vi "HFRR ADV v013 new software.vi"() -> ()   [LabVIEW 2025] (continued)
                              }
                              frame #3 {
                                n2582 = Wait (ms)(milliseconds to wait=u32 1500) -> ()  [unwired: 1 out]
                              }
                              frame #4 {
                                n2583 = local write "Command"("HE;0" ("Command")) -> ()
                              }
                            }
                          }
                        }
                      }
                      frame True {
                      }
                    }
                    n2584 = local write "String 14"("Test will autostart once parameters reach the set value." ("String 14")) -> ()
                  }
                  frame True {
                    (unwired) FALSE ("Visible")
                    n2585 = property on="Stroke 2" class="DigNum (strict)"("Visible"=TRUE) -> ()  [unwired: 2 in, 2 out]
                    n2586 = property on="STOP 2" class="Bool (strict)"("Disabled"=u8 2) -> ()  [unwired: 2 in, 2 out]
                    n2587 = local write "String 14"(" Running....." ("String 14")) -> ()
                    n2588 = property on="Heater Button" class="Bool (strict)"("DisabledEnum"=T17."Disabled and Grayed Out" ("Disabled")) -> ()  [unwired: 2 in, 2 out]
                    n2589 = property on="Humidity" class="Bool (strict)"("DisabledEnum"=T17."Disabled and Grayed Out" ("Disabled")) -> ()  [unwired: 2 in, 2 out]
                    n2590 = case shown="True" "Start Time" {
                      selector: "Start Time" -> [_ w3109]
                      frame False {
                      }
                      frame True {
                        n2591 = Not(x=w3109) -> (.not. x?=w3108:bool)
                        n2592 = local write "Start Time"(w3108) -> ()
                        n2593 = local read "EVENT LOG"() -> (w3110:string)
                        n2594 = call "Event Log.vi"("Content"="Test in progress", "EVENT LOG"=w3110) -> ("EVENT LOG"=w3112:string)  [unwired: 8 in, 1 out]
                        n2595 = local write "EVENT LOG"(w3112) -> ()
                      }
                    }
                    n2596 = disable-structure shown="Enabled" {
                      disable-tunnel: [w3101 w3107] -> w3090
                      frame Disabled {
                        n2597 = local read "Set Hz"() -> (w3104:dbl)
                        n2598 = call <vilib>:"Uniform White Noise Waveform.vi"() -> ("signal out"=w3103:waveform(dbl))  [unwired: 10 in, 1 out]
                        n2599 = Random Number (0-1)() -> (number: 0 to 1=w3100:dbl)
                        n2600 = Add(x=w3104, y=w3103) -> (x+y=w3102:waveform(dbl))
                        n2601 = Multiply(x=ext 0.01 ("y"), y=w3100) -> (x*y=w3098:ext)
                        n2602 = Multiply(x=w3102, y=w3098) -> (x*y=w3101:waveform(ext))
                      }
                      frame Enabled {
                        n2603 = call-poly <vilib>:"Random Number (Range).vi"("lower bound (0)"=49.89, "upper bound (100)"=50.8) -> ("number"=w3107:dbl)  [unwired: 9 in]
                      }
                    }
                    "StartFlg" <- TRUE ("StartFlg")
                  }
                }
                n2604 = case shown="True" w3061 {
                  frame False {
                  }
                  frame True {
                    n2605 = local write "clk"(10.0 ("clk")) -> ()
                    n2606 = Get Date/Time In Seconds() -> (seconds since 1Jan1904=w3115:timestamp)
                    n2607 = To Double Precision Float(number=w3115) -> (double precision float=w3113:dbl)
                    n2608 = local write "acq timer"(w3113) -> ()
                    n2609 = local write "act save time"(w3113) -> ()
                  }
                }
                n2610 = call "Elapsed Time"("Time Target (s)"="Countdown", "Reset"=w3050) -> ("Elapsed Time (s)"=w3055:dbl, "Time has Elapsed"=w3053:bool)  [unwired: 10 in, 6 out]
                "Countdown 2" <- w3055
                n2611 = Subtract(x=w3055, y=2.0) -> (x-y=w3058:dbl)
                n2612 = Less?(x=w3058, y="Countdown") -> (x < y?=w3056:bool)
                n2613 = And(x=w3056, y=w3053) -> (x .and. y?=w3052:bool)
                n2614 = case shown="True" w3052 {
                  frame False {
                  }
                  frame True {
                    (unwired) dbl[] [] ("History Data")
                    n2615 = local write "Engage"(FALSE ("Engage")) -> ()
                    n2616 = local write "RUN"(TRUE ("RUN")) -> ()
                    n2617 = local read "Humidity ( %RH )"() -> (→"Rh Before":dbl)
                  }
                }
                n2618 = local read "Test \nStatus"() -> (w3048:bool)
                n2619 = Select(t=w3046, s=w3048, f=0.0) -> (s? t:f=w3047:dbl)
                n2620 = local write "Frequency ( Hz )"(w3047) -> ()
              }
              frame #1 {
                w3138 = 1000000.0 ("x")
                # "HC;1/0\nST;VALUE"
                # "Elapsed time\ncof\nstroke\nAir temp\nTemp\nHumidity"
                # "acq timer\n\nact save time"
                # "convert to microseconds"
                n2621 = local read "COUNT"() -> (w3121:i32)
                n2622 = local read "Rate"() -> (w3134:dbl)
                n2623 = Divide(x=w3138, y=w3134) -> (x/y=w3139:dbl)
                n2624 = Greater Or Equal?(x=w3121, y=250) -> (x >= y?=w3120:bool)
                n2625 = Get Date/Time In Seconds() -> (seconds since 1Jan1904=w3141:timestamp)
                n2626 = case shown="True" w3120 {
                  frame False {
                    n2627 = local read "COUNT"() -> (w3142:i32)
                    n2628 = Increment(x=w3142) -> (x+1=w3143:i32)
                    n2629 = local write "COUNT"(w3143) -> ()
                  }
                  frame True {
                    n2630 = local write "COUNT"(0 ("COUNT")) -> ()
                  }
                }
                n2631 = local read "Samplingtime 2"() -> (w3119:dbl)
                n2632 = local read "act save time"() -> (w3136:dbl)
                n2633 = Divide(x=w3139, y=w3138) -> (x/y=w3137:dbl)
                n2634 = To Double Precision Float(number=w3141) -> (double precision float=w3130:dbl)
                n2635 = Add(x=w3136, y=w3119) -> (x+y=w3135:dbl)
                n2636 = local read "acq timer"() -> (w3140:dbl)
                n2637 = local read "COUNT"() -> (w3123:i32)
                n2638 = Greater Or Equal?(x=w3130, y=w3135) -> (x >= y?=w3118:bool)
                n2639 = Multiply(x=w3137, y=w3123) -> (x*y=w3129:dbl)
                n2640 = Subtract(x=w3130, y=w3140) -> (x-y=w3132:dbl)
                n2641 = local read "Save"() -> (w3133:bool)
                n2642 = Add(x=w3132, y=w3129) -> (x+y=w3116:dbl)
                "Elapsed time 3" <- w3116
                n2643 = And(x=w3118, y=w3133) -> (x .and. y?=w3131:bool)
                n2644 = Divide(x=w3116, y=60.0) -> (x/y=w3127:dbl)
                n2645 = local read "Test \nStatus"() -> (w3117:bool)
                n2646 = local read "clk"() -> (w3124:dbl)
                n2647 = Equal?(x=w3124, y=10.0) -> (x = y?=w3126:bool)
                n2648 = case shown="True" w3131 {
                  tunnel: w3130 -> [_ w3254]
                  tunnel: [FALSE ("Boolean 2") TRUE ("Boolean 2")] -> _
                  frame False {
                  }
                  frame True {
                    w3208 = ";" ("Substring")
                    # "Pid out/\nFreq response value"
                    n2649 = local write "act save time"(w3254) -> ()
                    n2650 = local read "FILE"() -> (w3202:string)
                    n2651 = call "file check.vi"("file name in"=w3202) -> ("error out"=w3205:errorcluster, "file name out"=w3200:string)  [unwired: 9 in]
                    n2652 = local read "LVDT STROKE"() -> (w3197:dbl)
                    n2653 = local read "Add up Stroke"() -> (w3195:dbl)
                    n2654 = call "FILE PATH CREATION.vi"("error in"=w3205, "FILE NAME :"=w3200) -> ("FILE OUT"=w3203:path)  [unwired: 8 in, 1 out]
                    n2655 = Concatenate Strings(w3200, ".dgf" ("Substring")) -> (w3204:string)
                    n2656 = Subtract(x=w3197, y=w3195) -> (x-y=w3196:dbl)
                    n2657 = Absolute Value(x=w3196) -> (abs(x)=w3194:dbl)
                    n2658 = local read "FF 2"() -> (→"Frictional Force ( N )" →"Frictional Force ( N )":dbl)
                    n2659 = Build Path(base path=w3203, name or relative path=w3204) -> (appended path=w3199:path)
                    n2660 = local read "COF 2"() -> (w3213:dbl)
                    "cof" <- w3213
                    "Coefficient of Friction" <- w3213
                    "COF 4" <- w3213
                    "Coefficient of Friction" <- w3213
                    n2661 = local read "TEMP"() -> (w3216:dbl)
                    "Temp" <- w3216
                    "Temperature ( Deg C )" <- w3216
                    n2662 = local read "Humidity ( %RH )"() -> (w3215:dbl)
                    "Humidity ( %RH )" <- w3215
                    "Humidity ( %RH )" <- w3215
                    n2663 = local read "Frequency ( Hz )"() -> (w3222:dbl)
                    n2664 = call <vilib>:"Mean PtByPt.vi"("x"=w3194, "sample length"=10) -> ("mean"=w3193:dbl)  [unwired: 2 in, 1 out]
                    n2665 = local read "Elapsed time"() -> (w3247:dbl)
                    n2666 = local read "AIR TEMP"() -> (w3220:dbl)
                    n2667 = local read "PID-out"() -> (w3225:dbl)
                    n2668 = local write "Temperature ( Deg C )"(w3216) -> ()
                    n2669 = Number To Fractional String(number=w3193, width (-)=i16 9 ("precision (6)"), precision (6)=i16 6) -> (F-format string=w3240:string)  [unwired: 1 in]
                    n2670 = Number To Fractional String(number=w3220, width (-)=i16 9 ("precision (6)"), precision (6)=i16 3) -> (F-format string=w3239:string)  [unwired: 1 in]
                    n2671 = Number To Fractional String(number=w3216, width (-)=i16 9 ("precision (6)"), precision (6)=i16 3) -> (F-format string=w3236:string)  [unwired: 1 in]
                    n2672 = Number To Fractional String(number=w3215, width (-)=i16 9 ("precision (6)"), precision (6)=i16 3) -> (F-format string=w3233:string)  [unwired: 1 in]
                    n2673 = Number To Fractional String(number=0.0, width (-)=i16 9 ("precision (6)"), precision (6)=i16 3) -> (F-format string=w3230:string)  [unwired: 1 in]
                    n2674 = Number To Fractional String(number=w3225, width (-)=i16 9 ("precision (6)"), precision (6)=i16 3) -> (F-format string=w3226:string)  [unwired: 1 in]
                    n2675 = Number To Fractional String(number=w3222, width (-)=i16 9 ("precision (6)"), precision (6)=i16 3) -> (F-format string=w3221:string)  [unwired: 1 in]
                    n2676 = Number To Fractional String(number=w3213, width (-)=i16 9 ("precision (6)"), precision (6)=i16 6) -> (F-format string=w3248:string)  [unwired: 1 in]
                    n2677 = Number To Fractional String(number=w3247, width (-)=i16 14 ("precision (6)"), precision (6)=i16 3) -> (F-format string=w3249:string)  [unwired: 1 in]
                    n2678 = Bundle("y"=1.02, "mean"=w3193, "y"=0.98) -> (w3214:cluster{"y":dbl, "mean":dbl, "y":dbl})  [unwired: 1 in]
                    n2679 = Number To Fractional String(number="Ambient Humidity :", width (-)=i16 9 ("precision (6)"), precision (6)=i16 6) -> (F-format string=w3206:string)  [unwired: 1 in]
                    n2680 = local read "RUN"() -> (w3212:bool)
                    n2681 = case shown="True" w3212 {
                      tunnel: w3214 -> [_ w3259]
                      tunnel: w3193 -> [_ w3258]
                      tunnel: w3193 -> [_ w3256]
                      tunnel: w3193 -> [_ w3257]
                      frame False {
                      }
                      frame True {
                        "Stroke ( mm )" <- w3259
                        "Stroke ( mm )" <- w3259
                        "Stroke 4" <- w3258
                        "Stroke 3" <- w3256
                        "Stroke 2" <- w3257
                        "measured_stroke" <- w3256
                      }
                    }
                    n2682 = Concatenate Strings(w3249, w3208, w3248, w3208, w3240, w3208, w3239, w3208, w3236, w3208, w3233, w3208, w3230, w3208, w3226, w3208, w3221, w3208, w3206, "\r") -> (w3246:string)
                    n2683 = call <vilib>:"Write Characters To File.vi"("append to file? (new file:F)"=TRUE, "character string"=w3246, "file path (dialog if empty)"=w3199) -> ()  [unwired: 2 in, 1 out]
                    "refresh flag" <- TRUE ("refresh flag")
                  }
                }
                n2684 = case shown="True" w3117 {
                  tunnel: w3127 -> [_ w3153]
                  tunnel: w3132 -> [_ w3163]
                  tunnel: [0.0 w3159] -> _
                  tunnel: w3126 -> [_ w3158]
                  tunnel: [0.0 w3157] -> _
                  tunnel: w3116 -> [_ w3157]
                  tunnel: w3130 -> [w3146 _]
                  frame False {
                    n2685 = local write "acq timer"(w3146) -> ()
                    n2686 = local write "Test Duration Status"(0.0 ("Test Duration Status")) -> ()
                  }
                  frame True {
                    n2687 = local read "Set Hz"() -> (w3160:dbl)
                    n2688 = local write "Elapsed time"(w3153) -> ()
                    n2689 = local read "test time"() -> (w3152:dbl)
                    n2690 = Multiply(x=w3163, y=w3160) -> (x*y=w3162:dbl)
                    n2691 = case shown="False" w3158 {
                      tunnel: w3162 -> [w3164 _]
                      tunnel: [w3164 1.0] -> w3159
                      frame False {
                        n2692 = local write "Cycles elapsed"(w3164) -> ()
                      }
                      frame True {
                      }
                    }
                    n2693 = Greater?(x=w3153, y=w3152) -> (0:w3161:bool)
                    n2694 = Subtract(x=w3152, y=w3153) -> (x-y=w3151:dbl)
                    "time" <- w3151
                    n2695 = Multiply(x=w3151, y=60.0) -> (x*y=w3150:dbl)
                    n2696 = local write "Time Remaining"(w3150) -> ()
                    n2697 = local write "Remaining Time"(w3150) -> ()
                    n2698 = case shown="True" w3161 {
                      frame False {
                      }
                      frame True {
                        n2699 = stacked-sequence {
                          frame #0 {
                            w3169 = T17."Enabled" ("Disabled")
                            w3168 = FALSE ("TEST FILE NAM,E SAVED")
                            w3170 = "" ("FILE")
                            w3171 = TRUE ("Visible")
                            n2700 = local write "Humidity"(FALSE ("Humidity")) -> ()
                            n2701 = local write "RUN"(FALSE ("OK Button 2")) -> ()
                            n2702 = local write "Heater Button"(FALSE ("Heater Button")) -> ()
                            n2703 = local write "Auto Start Test"(FALSE ("Auto Start Test")) -> ()
                            n2704 = local write "TestCompFlg"(TRUE ("StpFlg")) -> ()
                            n2705 = local read "Humidity ( %RH )"() -> (→"Rh After":dbl)
                            n2706 = property on="STOP 2" class="Bool (strict)"("Disabled"=u8 0) -> ()  [unwired: 2 in, 2 out]
                            n2707 = local read "EVENT LOG"() -> (w3176:string)
                            n2708 = call "Event Log.vi"("Content"="Test Completed", "EVENT LOG"=w3176) -> ("EVENT LOG"=w3175:string)  [unwired: 8 in, 1 out]
                            n2709 = property on="RUN" class="Bool (strict)"("Visible"=w3171) -> ()  [unwired: 2 in, 2 out]
                            n2710 = property on="Auto Start Test" class="Bool (strict)"("Visible"=w3171) -> ()  [unwired: 2 in, 2 out]
                            n2711 = local write "Batch Ref Num :"(w3170) -> ()
                            n2712 = local write "FILE"(w3170) -> ()
                            n2713 = local write "EVENT LOG"(w3175) -> ()
                            n2714 = local write "TEST FILE NAM,E SAVED"(w3168) -> ()
                            n2715 = local write "Fuel Discription :"(w3170) -> ()
                            n2716 = local write "START TEMP"(w3168) -> ()
                            n2717 = local write "Remarks :"(w3170) -> ()
                            n2718 = local write "Main Dashboard Buttons"(T1."Imaging" ("Main Dashboard Buttons")) -> ()
                            n2719 = local write "Main Tab"(T2."Adv Scar" ("Main Tab")) -> ()
                            n2720 = property on="FRICVALZ 2" class="Bool (strict)"("DisabledEnum"=w3169) -> ()  [unwired: 2 in, 2 out]
                            n2721 = property on="FRICVALZ 3" class="Bool (strict)"("DisabledEnum"=w3169) -> ()  [unwired: 2 in, 2 out]
                            n2722 = property on="FRICVALZ 4" class="Bool (strict)"("DisabledEnum"=w3169) -> ()  [unwired: 2 in, 2 out]
                          }
                          frame #1 {
                            n2723 = Wait (ms)(milliseconds to wait=u32 1500) -> ()  [unwired: 1 out]
                          }
                          frame #2 {
                            n2724 = local write "Command"("VC;0") -> ()
                          }
                          frame #3 {
                            n2725 = Wait (ms)(milliseconds to wait=u32 1500) -> ()  [unwired: 1 out]
                          }
                          frame #4 {
                            n2726 = local write "Command"("VC;0") -> ()
                          }
                          frame #5 {
                            n2727 = Wait (ms)(milliseconds to wait=u32 1500) -> ()  [unwired: 1 out]
                          }
                          frame #6 {
                            n2728 = local write "Command"("ST;0") -> ()
                          }
                          frame #7 {
                            n2729 = local write "measured_stroke"(0.0 ("measured_stroke")) -> ()
                            n2730 = Wait (ms)(milliseconds to wait=u32 1500) -> ()  [unwired: 1 out]
                          }
                          frame #8 {
                            n2731 = local write "Command"("HE;0") -> ()
                          }
                        }
                      }
                    }
                    n2732 = Divide(x=w3153, y=w3152) -> (x/y=w3156:dbl)
                    n2733 = Multiply(x=w3156, y=100.0) -> (x*y=w3154:dbl)
                    n2734 = local write "Test Duration Status"(w3154) -> ()
                  }
                }
              }
              frame #2 {
                n2735 = case shown="True" "Heater Button" {
                  tunnel: [0.0 ("output") w3282] -> w3260
                  frame False {
                    w3263 = TRUE ("tmpchk")
                    n2736 = local read "TEMP"() -> (w3264:dbl)
                    n2737 = local write "Temp ini"(w3264) -> ()
                    n2738 = local write "Reset 4"(w3263) -> ()
                    n2739 = local write "tmpchk"(w3263) -> ()
                    n2740 = local write "reinit"(TRUE ("reinit")) -> ()
                    n2741 = local write "manual temp log"(TRUE ("manual temp log")) -> ()
                  }
                  frame True {
                    # "Logic to turn off\nthe heater when \ntemp is not rising.\nTime - 60 sec\nDelta t- 5°c"
                    n2742 = local read "Temp ini"() -> (w3271:dbl)
                    n2743 = local read "Auto Start Test"() -> (w3267:bool)
                    n2744 = Less?(x=w3271, y=53.0) -> (x < y?=w3269:bool)
                    n2745 = case shown="False" w3267 {
                      frame False {
                        n2746 = local read "Set Temp"() -> (w3291:dbl)
                        n2747 = local read "TEMP"() -> (w3290:dbl)
                        n2748 = Subtract(x=w3291, y=w3290) -> (x-y=w3289:dbl)
                        n2749 = Absolute Value(x=w3289) -> (abs(x)=w3288:dbl)
                        n2750 = Less?(x=w3288, y=0.5) -> (x < y?=w3286:bool)
                        n2751 = case shown="True" w3286 {
                          tunnel: "manual temp log" -> [_ w3292]
                          frame False {
                          }
                          frame True {
                            n2752 = case shown="True" w3292 {
                              selector: w3292 -> [_ w3293]
                              frame False {
                              }
                              frame True {
                                # "#Event log"
                                n2753 = Not(x=w3293) -> (.not. x?=w3294:bool)
                                n2754 = local write "manual temp log"(w3294) -> ()
                                n2755 = local read "EVENT LOG"() -> (w3297:string)
                                n2756 = call "Event Log.vi"("Content"="Target Temperature reached", "EVENT LOG"=w3297) -> ("EVENT LOG"=w3296:string)  [unwired: 8 in, 1 out]
                                n2757 = local write "EVENT LOG"(w3296) -> ()
                              }
                            }
                          }
                        }
                      }
                      frame True {
                        n2758 = local write "manual temp log"(TRUE ("manual temp log")) -> ()
                      }
                    }
                    n2759 = And(x="tmpchk", y=w3269) -> (x .and. y?=w3272:bool)
                    n2760 = case shown="True" w3272 {
                      frame False {
                      }
                      frame True {
                        n2761 = call "Elapsed Time8"("Time Target (s)"=300.0, "Reset"="Reset 4") -> ("Time has Elapsed"=w3299:bool)  [unwired: 10 in, 7 out]
                        n2762 = flat-sequence {
                          tunnel: w3299 -> [_]
                          frame #0 {
                            n2763 = local write "Reset 4"(FALSE ("Reset 4")) -> ()
                          }
                        }
                        n2764 = case shown="True" w3299 {
                          frame False {
                          }
                          frame True {
                            n2765 = local read "Temp ini"() -> (w3306:dbl)
                            n2766 = Add(x=w3306, y=5.0) -> (x+y=w3304:dbl)
                            n2767 = local read "TEMP"() -> (w3307:dbl)
                            n2768 = Greater?(x=w3307, y=w3304) -> (0:w3305:bool)
                            n2769 = case shown="False" w3305 {
                              frame False {
                                n2770 = local write "Heater Button"(FALSE ("Heater Button")) -> ()
                              }
                              frame True {
                                n2771 = local write "tmpchk"(FALSE ("tmpchk")) -> ()
                              }
                            }
                          }
                        }
                      }
                    }
                    n2772 = local read "Set Temp"() -> (w3280:dbl)
                    n2773 = local read "TEMP"() -> (w3274:dbl)
                    n2774 = call-poly <vilib>:"PID.vi"("reinitialize? (F)"="reinit", "dt (s)"=-1.0, "process variable"=w3274, "setpoint"=w3280) -> ("output"=w3277:dbl)  [unwired: 6 in, 1 out]
                    n2775 = Subtract(x=w3280, y=w3274) -> (x-y=w3281:dbl)
                    n2776 = Add(x=w3280, y=0.5) -> (x+y=w3278:dbl)
                    n2777 = Greater Or Equal?(x=w3274, y=w3278) -> ()  [unwired: 1 out]
                    n2778 = Select(t=0.0, s=FALSE, f=w3277) -> (s? t:f=w3276:dbl)
                    "PID output" <- w3276
                    n2779 = flat-sequence {
                      tunnel: w3276 -> [w3310]
                      tunnel: [w3310] -> w3282
                      frame #0 {
                        n2780 = local write "reinit"(FALSE ("reinit")) -> ()
                      }
                    }
                    n2781 = Bundle(w3281, "output"=w3276, "TEMP"=w3274) -> ()  [unwired: 1 in, 1 out]
                  }
                }
                "PID-out" <- w3260
              }
              frame #3 {
                n2782 = local read "TEMP"() -> (w3312:dbl)
                n2783 = Greater Or Equal?(x=w3312, y="Set Temp 2") -> (x >= y?=w3317:bool)
                n2784 = case shown="True" w3317 {
                  tunnel: [FALSE TRUE] -> w3315
                  frame False {
                  }
                  frame True {
                  }
                }
                "Status 13" <- w3315
                n2785 = And(x=w3315, y="trip1 8") -> (x .and. y?=w3314:bool)
                n2786 = case shown="True" w3314 {
                  frame False {
                    n2787 = local write "Heater Trip Temp"(TRUE ("Heater Trip Temp")) -> ()
                  }
                  frame True {
                    w3320 = FALSE ("OK Button 2")
                    n2788 = case shown="True" "Heater Trip Temp" {
                      selector: "Heater Trip Temp" -> [_ w3322]
                      frame False {
                      }
                      frame True {
                        n2789 = Not(x=w3322) -> (.not. x?=w3321:bool)
                        n2790 = local read "EVENT LOG"() -> (w3325:string)
                        n2791 = local write "Heater Trip Temp"(w3321) -> ()
                        n2792 = call "Event Log.vi"("Content"="Heater Trip", "EVENT LOG"=w3325) -> ("EVENT LOG"=w3324:string)  [unwired: 8 in, 1 out]
                        n2793 = local write "EVENT LOG"(w3324) -> ()
                      }
                    }
                    n2794 = local write "RUN"(w3320) -> ()
                    n2795 = property on="Auto Start Test" class="Bool (strict)"("Value"=w3320) -> ()  [unwired: 2 in, 2 out]
                    n2796 = local write "Heater Button"(w3320) -> ()
                  }
                }
              }
            }
            n2797 = case shown="False" w3041 {
              frame False {
                n2798 = disable-structure shown="Disabled" {
                  frame Disabled {
                    n2799 = stacked-sequence {
                      frame #0 {
                        n2800 = local write "RUN"(FALSE ("OK Button 2")) -> ()
                      }
                      frame #1 {
                      }
                    }
                  }
                  frame Enabled {
                  }
                }
              }
              frame True {
              }
            }
          }
        }
        n2801 = local read "airtempflg"() -> (w2833:bool)
        n2802 = Or(x=w2833, y=w2831) -> (x .or. y?=w2834:bool)
        n2803 = Insert Into Array(array=string[] ["Air Temperature has reached set value,", "Humidity has reached set value,", "Sample Temperaturehas reached set value,", ""], index=0, new element="") -> (w2819:string[])
        n2804 = Build Array(w2824, w2823, w2822) -> (w2820:i32[])
        n2805 = disable-structure shown="Disabled" {
          disable-tunnel: w2834 -> [w2911 _]
          disable-tunnel: w2829 -> [w2910 _]
          disable-tunnel: w2827 -> [w2909 _]
          frame Disabled {
            n2806 = Compound Arithmetic op=AND(w2911, w2910, w2909) -> ()  [unwired: 1 out]
            n2807 = case shown="True" {
              selector: _ -> [_ _]
              frame False {
              }
              frame True {
                w2912 = FALSE ("autostrtflg")
                n2808 = local write "RUN"(TRUE ("RUN")) -> ()
                n2809 = local write "autostrtflg"(w2912) -> ()
                n2810 = local write "autostart"(w2912) -> ()
                n2811 = local write "String 14"(" Running....." ("String 14")) -> ()
              }
            }
          }
          frame Enabled {
          }
        }
        n2812 = for {
          tunnel: w2820 -> [w2962] mode=indexing
          tunnel: w2819 -> [w2961]
          shift-right: [w2958] -> w2818
          shift-left: "" -> [w2960]
          n2813 = Index Array(array=w2961, index=w2962) -> (element=w2959:string)
          n2814 = Concatenate Strings(w2959, w2960) -> (w2958:string)
        }
        n2815 = local write "autostart 2"(w2818) -> ()
        n2816 = local read "Reset Graph"() -> (w2807:bool)
        n2817 = case shown="True" w2807 {
          selector: w2807 -> [_ w2861]
          frame False {
          }
          frame True {
            w2875 = 0.0 ("X Scale.Range:Maximum")
            n2818 = Not(x=w2861) -> (.not. x?=w2860:bool)
            n2819 = local write "Reset Graph"(w2860) -> ()
            n2820 = property on="Electrical Contact Resistance ( % )" class="WFChart (strict)"("XScale.Maximum"=600.0 ("X Scale.Range:Maximum"), "XScale.Minimum"=0.0 ("X Scale.Range:Minimum"), "YScale.Maximum"=100.0 ("Y Scale.Range:Maximum"), "YScale.Minimum"=0.0 ("Y Scale.Range:Minimum")) -> ()  [unwired: 2 in, 2 out]
            n2821 = property on="Frictional Force ( N )" class="WFChart (strict)"("XScale.Maximum"=600.0 ("X Scale.Range:Maximum"), "XScale.Minimum"=0.0 ("X Scale.Range:Minimum"), "YScale.Maximum"=100.0 ("Y Scale.Range:Maximum"), "YScale.Minimum"=0.0 ("Y Scale.Range:Minimum")) -> ()  [unwired: 2 in, 2 out]
            n2822 = property on="Temperature ( Deg C )" class="WFChart (strict)"("XScale.Maximum"=600.0 ("X Scale.Range:Maximum"), "XScale.Minimum"=0.0 ("X Scale.Range:Minimum"), "YScale.Maximum"=100.0 ("Y Scale.Range:Maximum"), "YScale.Minimum"=0.0 ("Y Scale.Range:Minimum")) -> ()  [unwired: 2 in, 2 out]
            n2823 = property on="Humidity ( %RH )" class="WFChart (strict)"("XScale.Maximum"=600.0 ("X Scale.Range:Maximum"), "XScale.Minimum"=0.0 ("X Scale.Range:Minimum"), "YScale.Maximum"=100.0 ("Y Scale.Range:Maximum"), "YScale.Minimum"=0.0 ("Y Scale.Range:Minimum")) -> ()  [unwired: 2 in, 2 out]
            n2824 = property on="Stroke ( mm )" class="WFChart (strict)"("XScale.Maximum"=600.0 ("X Scale.Range:Maximum"), "XScale.Minimum"=0.0 ("X Scale.Range:Minimum"), "YScale.Maximum"=100.0 ("Y Scale.Range:Maximum"), "YScale.Minimum"=0.0 ("Y Scale.Range:Minimum")) -> ()  [unwired: 2 in, 2 out]
            n2825 = property on="Coefficient of Friction" class="WFChart (strict)"("XScale.Maximum"=600.0 ("X Scale.Range:Maximum"), "XScale.Minimum"=0.0 ("X Scale.Range:Minimum"), "YScale.Maximum"=100.0 ("Y Scale.Range:Maximum"), "YScale.Minimum"=0.0 ("Y Scale.Range:Minimum")) -> ()  [unwired: 2 in, 2 out]
            n2826 = property on="Electrical Contact Resistance ( % )" class="WFChart (strict)"("XScale.Minimum"=0.0 ("X Scale.Range:Minimum"), "XScale.Maximum"=600.0 ("X Scale.Range:Maximum"), "YScale.Minimum"=0.0 ("Y Scale.Range:Minimum"), "YScale.Maximum"=100.0 ("Y Scale.Range:Maximum")) -> ()  [unwired: 2 in, 2 out]
            n2827 = property on="Temperature ( Deg C )" class="WFChart (strict)"("XScale.Minimum"=0.0 ("X Scale.Range:Minimum"), "XScale.Maximum"=600.0 ("X Scale.Range:Maximum"), "YScale.Minimum"=0.0 ("Y Scale.Range:Minimum"), "YScale.Maximum"=100.0 ("Y Scale.Range:Maximum")) -> ()  [unwired: 2 in, 2 out]
            n2828 = property on="Coefficient of Friction" class="WFChart (strict)"("XScale.Minimum"=0.0 ("X Scale.Range:Minimum"), "XScale.Maximum"=600.0 ("X Scale.Range:Maximum"), "YScale.Maximum"=1.0 ("X Scale.Range:Minimum"), "YScale.Minimum"=0.0 ("X Scale.Range:Minimum")) -> ()  [unwired: 2 in, 2 out]
            n2829 = property on="Frictional Force ( N )" class="WFChart (strict)"("XScale.Maximum"=600.0 ("X Scale.Range:Maximum"), "XScale.Minimum"=w2875, "YScale.Maximum"=10.0 ("Y Scale.Range:Maximum"), "YScale.Minimum"=w2875) -> ()  [unwired: 2 in, 2 out]
            n2830 = property on="Stroke ( mm )" class="WFChart (strict)"("XScale.Maximum"=600.0 ("X Scale.Range:Maximum"), "XScale.Minimum"=0.0 ("X Scale.Range:Minimum"), "YScale.Maximum"=100.0 ("Y Scale.Range:Maximum"), "YScale.Minimum"=0.0 ("Y Scale.Range:Minimum")) -> ()  [unwired: 2 in, 2 out]
            n2831 = property on="Humidity ( %RH )" class="WFChart (strict)"("XScale.Maximum"=600.0 ("X Scale.Range:Maximum"), "XScale.Minimum"=0.0 ("X Scale.Range:Minimum"), "YScale.Maximum"=100.0 ("Y Scale.Range:Maximum"), "YScale.Minimum"=0.0 ("Y Scale.Range:Minimum")) -> ()  [unwired: 2 in, 2 out]
          }
        }
      }
      frame "Compare Files" {
        # "Elapsed time\ncof\nstroke\nAir temp\nTemp\nHumidity"
        n2832 = case shown="True" "RSTV1 2" {
          frame False {
          }
          frame True {
            n2833 = property on="Humidity ( %RH )" class="XYGraph (strict)"("Y Scale.Display Format:Precision"=u8 0 ("Y Scale.Format & Precision:Precision")) -> ()  [unwired: 2 in, 2 out]
            n2834 = property on="Humidity ( %RH )" class="XYGraph (strict)"("X Scale.Range:Minimum"=0.0, "X Scale.Range:Maximum"=75.0, "Y Scale.Range:Minimum"=48.0, "Y Scale.Range:Maximum"=58.0) -> ()  [unwired: 2 in, 2 out]
          }
        }
        n2835 = case shown="True" "RST CP 2" {
          frame False {
          }
          frame True {
            n2836 = property on="XY Graph 13" class="XYGraph (strict)"("Y Scale.Display Format:Precision"=u8 0 ("Y Scale.Format & Precision:Precision")) -> ()  [unwired: 2 in, 2 out]
            n2837 = property on="XY Graph 13" class="XYGraph (strict)"("X Scale.Range:Minimum"=0.0, "X Scale.Range:Maximum"=75.0, "Y Scale.Range:Minimum"=0.0, "Y Scale.Range:Maximum"=100.0) -> ()  [unwired: 2 in, 2 out]
          }
        }
        n2838 = case shown="True" "RST CP" {
          frame False {
          }
          frame True {
            n2839 = property on="Sample Temperature ( °C )" class="XYGraph (strict)"("Y Scale.Display Format:Precision"=u8 2 ("Y Scale.Format & Precision:Precision")) -> ()  [unwired: 2 in, 2 out]
            n2840 = property on="Sample Temperature ( °C )" class="XYGraph (strict)"("X Scale.Range:Minimum"=0.0, "X Scale.Range:Maximum"=75.0, "Y Scale.Range:Minimum"=58.0, "Y Scale.Range:Maximum"=62.0) -> ()  [unwired: 2 in, 2 out]
          }
        }
        n2841 = case shown="True" "RSTV1 3" {
          frame False {
          }
          frame True {
            n2842 = property on="Air Temperature  ( °C )" class="XYGraph (strict)"("Y Scale.Display Format:Precision"=u8 2 ("Y Scale.Format & Precision:Precision")) -> ()  [unwired: 2 in, 2 out]
            n2843 = property on="Air Temperature  ( °C )" class="XYGraph (strict)"("X Scale.Range:Minimum"=0.0 ("Y Scale.Range:Minimum"), "X Scale.Range:Maximum"=75.0 ("Y Scale.Range:Maximum"), "Y Scale.Range:Minimum"=20.0 ("X Scale.Range:Minimum"), "Y Scale.Range:Maximum"=26.0 ("X Scale.Range:Maximum")) -> ()  [unwired: 2 in, 2 out]
          }
        }
        n2844 = case shown="True" "RSTV1 4" {
          frame False {
          }
          frame True {
            n2845 = property on="Stroke ( mm )" class="XYGraph (strict)"("Y Scale.Display Format:Precision"=u8 2 ("Y Scale.Format & Precision:Precision")) -> ()  [unwired: 2 in, 2 out]
            n2846 = property on="Stroke ( mm )" class="XYGraph (strict)"("X Scale.Range:Minimum"=0.0 ("Y Scale.Range:Maximum"), "X Scale.Range:Maximum"=75.0 ("X Scale.Range:Minimum"), "Y Scale.Range:Minimum"=0.98, "Y Scale.Range:Maximum"=1.02) -> ()  [unwired: 2 in, 2 out]
          }
        }
        n2847 = case shown="True" "rstv2" {
          frame False {
          }
          frame True {
            n2848 = property on="Coefficient Of Friction" class="XYGraph (strict)"("Y Scale.Display Format:Precision"=u8 3 ("Y Scale.Format & Precision:Precision")) -> ()  [unwired: 2 in, 2 out]
            n2849 = property on="Coefficient Of Friction" class="XYGraph (strict)"("X Scale.Range:Minimum"=0.0 ("Y Scale.Range:Maximum"), "X Scale.Range:Maximum"=75.0, "Y Scale.Range:Minimum"=0.0, "Y Scale.Range:Maximum"=1.0 ("X Scale.Range:Minimum")) -> ()  [unwired: 2 in, 2 out]
          }
        }
        n2850 = case shown="True" "RST CP 3" {
          frame False {
          }
          frame True {
            n2851 = property on="Air Temp ( °C ) vs Humidity ( % RH )" class="XYGraph (strict)"("X Scale.Range:Minimum"=18.0, "X Scale.Range:Maximum"=28.0 ("X Scale.Range:Minimum"), "Y Scale.Range:Minimum"=30.0 ("X Scale.Range:Minimum"), "Y Scale.Range:Maximum"=70.0 ("X Scale.Range:Minimum")) -> ()  [unwired: 2 in, 2 out]
          }
        }
        n2852 = case shown="True" "OPEN 1" {
          frame False {
          }
          frame True {
            (unwired) 0  # existing file
            w3601 = "Choose a datalog file to open"  # prompt
            n2853 = local write "OPEN 1"(FALSE ("OPEN 1")) -> ()
            n2854 = String To Path(string="C:\\LAB-IQ\\Data\\") -> (path=w3586:path)
            n2855 = File Dialog(6:"*.dgf" ("pattern"), 7:w3601, 11:w3586) -> (0:w3584:errorcluster, 3:w3592:path)  [unwired: 4 in, 2 out]
            n2856 = Unbundle(w3584) -> ()  [unwired: 3 out]
            n2857 = Strip Path(path=w3592) -> (name=w3591:string)  [unwired: 1 out]
            n2858 = Path To String(path=w3592) -> (string=w3587:string)
            "string1" <- w3587
            n2859 = Match Pattern(string=w3591, regular expression=".dgf") -> (before substring=→"String Control":string)  [unwired: 1 in, 3 out]
            n2860 = Match Pattern(string=w3587, regular expression=".dgf" ("substring (\"\")")) -> (before substring=w3597:string)  [unwired: 1 in, 3 out]
            n2861 = Concatenate Strings(w3597, ".duf" ("Substring")) -> (w3593:string)
            n2862 = String To Path(string=w3593) -> (path=w3598:path)
            n2863 = call <vilib>:"Read Characters From File.vi"("file path (dialog if empty)"=w3598, "start of read offset (chars.:0)"=60 ("start of read offset (chars.: 0)")) -> ("character string"=→"String Control 2":string)  [unwired: 4 in, 3 out]
          }
        }
        n2864 = case shown="True" "OPEN 2" {
          frame False {
          }
          frame True {
            (unwired) 0  # existing file
            w3619 = "Choose a datalog file to open"  # prompt
            n2865 = local write "OPEN 2"(FALSE ("OPEN 1")) -> ()
            n2866 = String To Path(string="C:\\LAB-IQ\\Data\\") -> (path=w3604:path)
            n2867 = File Dialog(6:"*.dgf" ("pattern"), 7:w3619, 11:w3604) -> (0:w3602:errorcluster, 3:w3610:path)  [unwired: 4 in, 2 out]
            n2868 = Unbundle(w3602) -> ()  [unwired: 3 out]
            n2869 = Strip Path(path=w3610) -> (name=w3608:string)  [unwired: 1 out]
            n2870 = Path To String(path=w3610) -> (string=w3605:string)
            "string1 2" <- w3605
            n2871 = Match Pattern(string=w3608, regular expression=".dgf") -> (before substring=→"String Control 3":string)  [unwired: 1 in, 3 out]
            n2872 = Match Pattern(string=w3605, regular expression=".dgf" ("substring (\"\")")) -> (before substring=w3616:string)  [unwired: 1 in, 3 out]
            n2873 = Concatenate Strings(w3616, ".duf" ("Substring")) -> (w3613:string)
            n2874 = String To Path(string=w3613) -> (path=w3611:path)
            n2875 = call <vilib>:"Read Characters From File.vi"("file path (dialog if empty)"=w3611, "start of read offset (chars.:0)"=60 ("start of read offset (chars.: 0)")) -> ("character string"=→"String Control 4":string)  [unwired: 4 in, 3 out]
          }
        }
        n2876 = case shown="True" "OPEN 3" {
          frame False {
          }
          frame True {
            (unwired) 0  # existing file
            w3637 = "Choose a datalog file to open"  # prompt
            n2877 = local write "OPEN 3"(FALSE ("OPEN 1")) -> ()
            n2878 = String To Path(string="C:\\LAB-IQ\\Data\\") -> (path=w3622:path)
            n2879 = File Dialog(6:"*.dgf" ("pattern"), 7:w3637, 11:w3622) -> (0:w3620:errorcluster, 3:w3628:path)  [unwired: 4 in, 2 out]
            n2880 = Unbundle(w3620) -> ()  [unwired: 3 out]
            n2881 = Strip Path(path=w3628) -> (name=w3626:string)  [unwired: 1 out]
            n2882 = Path To String(path=w3628) -> (string=w3623:string)
            "string1 3" <- w3623
            n2883 = Match Pattern(string=w3626, regular expression=".dgf") -> (before substring=→"String Control 5":string)  [unwired: 1 in, 3 out]
            n2884 = Match Pattern(string=w3623, regular expression=".dgf" ("substring (\"\")")) -> (before substring=w3633:string)  [unwired: 1 in, 3 out]
            n2885 = Concatenate Strings(w3633, ".duf" ("Substring")) -> (w3630:string)
            n2886 = String To Path(string=w3630) -> (path=w3634:path)
            n2887 = call <vilib>:"Read Characters From File.vi"("file path (dialog if empty)"=w3634, "start of read offset (chars.:0)"=60 ("start of read offset (chars.: 0)")) -> ("character string"=→"String Control 6":string)  [unwired: 4 in, 3 out]
          }
        }
        n2888 = case shown="True" "OPEN 4" {
          frame False {
          }
          frame True {
            (unwired) 0  # existing file
            w3655 = "Choose a datalog file to open"  # prompt
            n2889 = local write "OPEN 4"(FALSE ("OPEN 1")) -> ()
            n2890 = String To Path(string="C:\\LAB-IQ\\Data\\") -> (path=w3640:path)
            n2891 = File Dialog(6:"*.dgf" ("pattern"), 7:w3655, 11:w3640) -> (0:w3638:errorcluster, 3:w3646:path)  [unwired: 4 in, 2 out]
            n2892 = Unbundle(w3638) -> ()  [unwired: 3 out]
            n2893 = Strip Path(path=w3646) -> (name=w3644:string)  [unwired: 1 out]
            n2894 = Path To String(path=w3646) -> (string=w3641:string)
            "string1 4" <- w3641
            n2895 = Match Pattern(string=w3644, regular expression=".dgf") -> (before substring=→"String Control 7":string)  [unwired: 1 in, 3 out]
            n2896 = Match Pattern(string=w3641, regular expression=".dgf" ("substring (\"\")")) -> (before substring=w3651:string)  [unwired: 1 in, 3 out]
            n2897 = Concatenate Strings(w3651, ".duf" ("Substring")) -> (w3648:string)
            n2898 = String To Path(string=w3648) -> (path=w3652:path)
            n2899 = call <vilib>:"Read Characters From File.vi"("file path (dialog if empty)"=w3652, "start of read offset (chars.:0)"=60 ("start of read offset (chars.: 0)")) -> ("character string"=→"String Control 8":string)  [unwired: 4 in, 3 out]
          }
        }
      }
      frame "About" {
        # "Elapsed time\ncof\nstroke\nmean pos\nTemp\nHumidity"
        n2900 = disable-structure shown="Disabled" {
          frame Disabled {
            n2901 = case shown="True" "Export" {
              frame False {
              }
              frame True {
                w3677 = "                                      " ("string")
                w3679 = "\r"
                (unwired) i16 6 ("width (-)")
                w3756 = "\r"
                w3688 = "\r"
                n2902 = local write "Export"(FALSE ("Export")) -> ()
                n2903 = local read "String 29"() -> (w3725:string)
                n2904 = local read "String 34"() -> (w3713:string)
                n2905 = local read "String 35"() -> (w3708:string)
                n2906 = local read "String 37"() -> (w3704:string)
                n2907 = local read "String 36"() -> (w3701:string)
                n2908 = local read "String 38"() -> (w3698:string)
                n2909 = local read "String 39"() -> (w3695:string)
                n2910 = Match Pattern(string=w3725, regular expression=".dwm") -> (before substring=w3721:string)  [unwired: 1 in, 3 out]
                "before substring" <- w3721
                n2911 = local read "S 38"() -> (w3716:string)
                n2912 = local read "S 39"() -> (w3709:string)
                n2913 = local read "Temperature before test 2"() -> (w3745:dbl)
                n2914 = local read "Temperature after test 2"() -> (w3750:dbl)
                n2915 = local read "Humidity before test 2"() -> (w3731:dbl)
                n2916 = local read "Humidity after test 2"() -> (w3746:dbl)
                n2917 = local read "MWSD 2"() -> (w3742:dbl)
                n2918 = local read "WS1.4 2"() -> (w3758:dbl)
                n2919 = local read "HCF 2"() -> (w3754:dbl)
                n2920 = local read "AVP 2"() -> (w3743:dbl)
                n2921 = Concatenate Strings("1," ("string"), w3716) -> (w3715:string)
                n2922 = Concatenate Strings("2," ("string"), w3713) -> (w3712:string)
                n2923 = Concatenate Strings("3," ("string"), w3709) -> (w3711:string)
                n2924 = Concatenate Strings("4," ("string"), w3708) -> (w3707:string)
                n2925 = Concatenate Strings("5," ("string"), w3704) -> (w3705:string)
                n2926 = Concatenate Strings("6," ("string"), w3701) -> (w3702:string)
                n2927 = Concatenate Strings("7," ("string"), w3698) -> (w3699:string)
                n2928 = Concatenate Strings("8," ("string"), w3695) -> (w3696:string)
                n2929 = local read "Sample ID"() -> (w3763:string)
                n2930 = case shown="\"xlx\"" "Select File Type" {
                  tunnel: w3721 -> [w3766 w3768 w3770]
                  tunnel: [w3764 w3769 w3771] -> w3720
                  frame "xlx" {
                    n2931 = Concatenate Strings(w3766, ".xls" ("string")) -> (w3764:string)
                  }
                  frame "csv" {
                    n2932 = Concatenate Strings(w3768, ".csv" ("string")) -> (w3769:string)
                  }
                  frame "txt" {
                    n2933 = Concatenate Strings(w3770, ".txt" ("string")) -> (w3771:string)
                  }
                }
                n2934 = local read "Test Date"() -> (w3762:string)
                n2935 = local read "String 45"() -> (w3676:string)
                n2936 = local read "String 31"() -> (w3761:string)
                n2937 = local read "String 32"() -> (w3760:string)
                n2938 = local read "TITTLE"() -> (w3684:string)
                n2939 = Number To Fractional String(number=w3731, width (-)=i16 6, precision (6)=i16 2) -> (F-format string=w3730:string)  [unwired: 1 in]
                n2940 = Number To Fractional String(number=w3745, width (-)=i16 6, precision (6)=i16 2) -> (F-format string=w3751:string)  [unwired: 1 in]
                n2941 = Number To Fractional String(number=w3746, width (-)=i16 6, precision (6)=i16 2) -> (F-format string=w3744:string)  [unwired: 1 in]
                n2942 = Number To Fractional String(number=w3750, width (-)=i16 6, precision (6)=i16 2) -> (F-format string=w3749:string)  [unwired: 1 in]
                n2943 = Number To Fractional String(number=w3742, width (-)=i16 6, precision (6)=i16 2) -> (F-format string=w3740:string)  [unwired: 1 in]
                n2944 = Number To Fractional String(number=w3743, width (-)=i16 6, precision (6)=i16 2) -> (F-format string=w3741:string)  [unwired: 1 in]
                n2945 = Number To Fractional String(number=w3754, width (-)=i16 6, precision (6)=i16 2) -> (F-format string=w3755:string)  [unwired: 1 in]
                n2946 = Number To Fractional String(number=w3758, precision (6)=i16 2) -> (F-format string=w3759:string)  [unwired: 2 in]
                n2947 = local read "s.NO"() -> (w3678:string)
                n2948 = Concatenate Strings("=" ("string"), w3684) -> (w3683:string)
                n2949 = Concatenate Strings("S.No," ("string"), "                                       Parameters" ("string")) -> (w3689:string)
                n2950 = Concatenate Strings(w3756, w3715, w3730, w3756, w3712, w3751, w3756, w3711, w3744, w3756, w3707, w3749, w3756, w3705, w3740, w3756, w3702, w3741, w3756, w3699, w3755, w3756, w3696, w3759) -> (w3718:string)
                n2951 = Concatenate Strings(w3688, "," ("string"), w3676, w3678, w3677, w3760, w3763, w3677, w3761, w3762, w3688) -> (w3686:string)
                n2952 = local read "Tested by"() -> (w3692:string)
                n2953 = local read "String 33"() -> (w3693:string)
                n2954 = Concatenate Strings("," ("string"), "                                                                             " ("string")) -> (w3681:string)
                n2955 = Concatenate Strings(w3683, w3679, w3686, w3679, w3689, w3718, w3679, w3681, w3693, w3692) -> (→"export":string)
                n2956 = String To Path(string=w3720) -> (path=w3727:path)
                n2957 = local read "export"() -> (w3722:string)
                n2958 = call <vilib>:"Write Characters To File.vi"("append to file? (new file:F)"=FALSE, "character string"=w3722, "file path (dialog if empty)"=w3727) -> ()  [unwired: 2 in, 1 out]
              }
            }
          }
          frame Enabled {
          }
        }
        n2959 = case shown="True" "OK Button 17" {
          frame False {
          }
          frame True {
            (unwired) 0  # existing file
            w3980 = "Choose a datalog file to open"  # prompt
            n2960 = local write "OK Button 17"(FALSE ("OK Button 17")) -> ()
            n2961 = local read "String"() -> (w3975:string)
            n2962 = String To Path(string=w3975) -> (path=w3976:path)
            n2963 = File Dialog(6:"*.duf" ("pattern"), 7:w3980, 11:w3976) -> (0:w3967:errorcluster, 3:w3986:path)  [unwired: 4 in, 2 out]
            n2964 = Unbundle(w3967) -> ()  [unwired: 3 out]
            n2965 = Open/Create/Replace File "Open File"(file path (use dialog)=w3986) -> (refnum out=w3978:refnum<file>)  [unwired: 5 in, 2 out]
            n2966 = Strip Path(path=w3986) -> (name=w3984:string)  [unwired: 1 out]
            n2967 = Path To String(path=w3986) -> (string=w3969:string)
            n2968 = while {
              tunnel: w3978 -> [w3990]
              i -> [w3987]
              stop <- w3988 continue-if-true
              (unwired) TRUE ("line mode (F)")
              n2969 = Read from Text File "Read File"(file (use dialog)=w3990) -> (text=w3989:string)  [unwired: 3 in, 3 out]
              n2970 = local write "Numeric 16"(w3987) -> ()
              n2971 = String Length(string=w3989) -> (length=w3992:i32)
              n2972 = Greater?(x=w3992, y=1) -> (0:w3988:bool)
            }
            n2973 = local write "String 29"(w3969) -> ()
            n2974 = Search and Replace String(input string=w3969, search string=".duf", replace string=".dgf" ("replace string (\"\")")) -> (result string=→"String Indicator 4":string)  [unwired: 5 in, 3 out]
            n2975 = Match Pattern(string=w3984, regular expression=".dwm") -> (before substring=w3968:string)  [unwired: 1 in, 3 out]
            "String Indicator" <- w3968
            n2976 = Match Pattern(string=w3969, regular expression=".dwm" ("substring (\"\")")) -> (before substring=w3970:string)  [unwired: 1 in, 3 out]
            "String Indicator 3" <- w3970
            n2977 = local write "TITTLE 2"(w3968) -> ()
            n2978 = String To Path(string=w3970) -> (path=w3977:path)
            "path" <- w3977
            n2979 = call <vilib>:"Read Characters From File.vi"("file path (dialog if empty)"=w3977, "start of read offset (chars.:0)"=60 ("start of read offset (chars.: 0)")) -> ("character string"=→"String Indicator 2":string)  [unwired: 4 in, 3 out]
          }
        }
        n2980 = call <vilib>:"Query Available Printers.vi"() -> ("system configured printers"=w3669:string[])  [unwired: 9 in, 2 out]
        "System Configured Printers 2" <- w3669
        n2981 = local read "OK Button 16"() -> (w3666:bool)
        n2982 = case shown="True" "OK Button 16" {
          frame False {
          }
          frame True {
            n2983 = stacked-sequence {
              frame #0 {
                n2984 = local read "Numeric 16"() -> (w3994:i32)
                n2985 = local write "Numeric 10"(w3994) -> ()
              }
              frame #1 {
                n2986 = local read "S.NO"() -> (→"s.NO":string)
                n2987 = local read "String 29"() -> (w3998:string)
                n2988 = String To Path(string=w3998) -> (path=w3997:path)
                n2989 = Open/Create/Replace File "Open File"(file path (use dialog)=w3997) -> (refnum out=w3999:refnum<file>)  [unwired: 5 in, 2 out]
                n2990 = for {
                  N: 16 -> [_]
                  tunnel: w3999 -> [w4006]
                  i -> [w4002]
                  (unwired) TRUE ("line mode (F)")
                  n2991 = Read from Text File "Read File"(file (use dialog)=w4006) -> (text=w4000:string)  [unwired: 3 in, 3 out]
                  n2992 = Match Pattern(string=w4000, regular expression="(") -> (after substring=w4005:string)  [unwired: 1 in, 3 out]
                  n2993 = Match Pattern(string=w4005, regular expression=")") -> (before substring=w4001:string)  [unwired: 1 in, 3 out]
                  n2994 = case shown="1" w4002 {
                    tunnel: w4001 -> [w4007 w4008 _ _ w4009 w4010 w4011 w4013 w4015 w4017 w4019 w4021 w4023 w4025 _]
                    tunnel: w4000 -> [_ _ _ _ _ _ _ _ _ _ _ _ _ _ _]
                    frame 0 {
                      "TITTLE" <- w4007
                    }
                    frame 1 {
                      "Sample ID" <- w4008
                    }
                    frame 2 {
                    }
                    frame 3 {
                    }
                    frame 4 {
                      "Test Date" <- w4009
                    }
                    frame 5 {
                      "Tested by" <- w4010
                    }
                    frame 6 {
                      n2995 = Fract/Exp String To Number(string=w4011) -> (number=→"Humidity before test 2":dbl)  [unwired: 3 in, 1 out]
                    }
                    frame 7 {
                      n2996 = Fract/Exp String To Number(string=w4013) -> (number=→"Temperature before test 2":dbl)  [unwired: 3 in, 1 out]
                    }
                    frame 8 {
                      n2997 = Fract/Exp String To Number(string=w4015) -> (number=→"Humidity after test 2":dbl)  [unwired: 3 in, 1 out]
                    }
                    frame 9 {
                      n2998 = Fract/Exp String To Number(string=w4017) -> (number=→"Temperature after test 2":dbl)  [unwired: 3 in, 1 out]
                    }
                    frame 10 {
                      n2999 = Fract/Exp String To Number(string=w4019) -> (number=→"MWSD 2":dbl)  [unwired: 3 in, 1 out]
                    }
                    frame 11 {
                      n3000 = Fract/Exp String To Number(string=w4021) -> (number=→"AVP 2":dbl)  [unwired: 3 in, 1 out]
                    }
                    frame 12 {
                      n3001 = Fract/Exp String To Number(string=w4023) -> (number=→"HCF 2":dbl)  [unwired: 3 in, 1 out]
                    }
                    frame 13 {
                      n3002 = Fract/Exp String To Number(string=w4025) -> (number=→"WS1.4 2":dbl)  [unwired: 3 in, 1 out]
                    }
                    frame 14, Default {
                    }
                  }
                }
              }
              frame #2 {
              }
            }
            n3003 = local write "OK Button 16"(FALSE ("OK Button 13")) -> ()
          }
        }
        n3004 = Index Array(array=w3669, index="Select Printer 3") -> (element=w3671:string)
        "Selected Printer" <- w3671
        n3005 = case shown="True" w3666 {
          frame False {
          }
          frame True {
            n3006 = flat-sequence {
              frame #0 {
              }
              frame #1 {
                n3007 = Wait (ms)(milliseconds to wait=u32 100) -> ()  [unwired: 1 out]
              }
              frame #2 {
                n3008 = local write "OK Button 16"(FALSE ("Print 3")) -> ()
              }
            }
          }
        }
        n3009 = case shown="True" "Print" {
          tunnel: w3671 -> [_ w3963]
          frame False {
          }
          frame True {
            (unwired) i16 6 ("width (-)")
            (unwired) "TESTED BY : "
            (unwired) "TESTED DATE :"
            (unwired) "SAMPLE ID : "
            (unwired) "SAMPLE DESIGN : "
            w3921 = "\r"
            w3938 = "\r"
            # "add image"
            n3010 = local read "Sample ID"() -> (w3911:string)
            n3011 = local read "Tested by"() -> (w3914:string)
            n3012 = local read "String 34"() -> (w3901:string)
            n3013 = local read "String 45"() -> (w3881:string)
            n3014 = local read "String 35"() -> (w3896:string)
            n3015 = local read "String 37"() -> (w3894:string)
            n3016 = local read "String 32"() -> (w3916:string)
            n3017 = local read "String 36"() -> (w3891:string)
            n3018 = local read "String 31"() -> (w3915:string)
            n3019 = local read "Test Date"() -> (w3912:string)
            n3020 = local read "String 33"() -> (w3917:string)
            n3021 = local read "String 38"() -> (w3887:string)
            n3022 = local read "String 39"() -> (w3884:string)
            n3023 = local write "Print"(FALSE ("Print FF")) -> ()
            n3024 = local read "S 39"() -> (w3899:string)
            n3025 = local read "S 38"() -> (w3906:string)
            n3026 = local read "Temperature before test 2"() -> (w3937:dbl)
            n3027 = local read "Temperature after test 2"() -> (w3927:dbl)
            n3028 = local read "Humidity before test 2"() -> (w3952:dbl)
            n3029 = local read "Humidity after test 2"() -> (w3936:dbl)
            n3030 = local read "MWSD 2"() -> (w3941:dbl)
            n3031 = local read "WS1.4 2"() -> (w3919:dbl)
            n3032 = Concatenate Strings("2)" ("string"), w3901) -> (w3902:string)
            n3033 = Concatenate Strings("3)" ("string"), w3899) -> (w3900:string)
            n3034 = Concatenate Strings("1)" ("string"), w3906) -> (w3905:string)
            n3035 = Concatenate Strings("4)" ("string"), w3896) -> (w3897:string)
            n3036 = Concatenate Strings("5)" ("string"), w3894) -> (w3893:string)
            n3037 = Concatenate Strings("6)" ("string"), w3891) -> (w3890:string)
            n3038 = Concatenate Strings("7)" ("string"), w3887) -> (w3888:string)
            n3039 = Concatenate Strings("8)" ("string"), w3884) -> (w3885:string)
            n3040 = local read "HCF 2"() -> (w3923:dbl)
            n3041 = local read "AVP 2"() -> (w3940:dbl)
            n3042 = local read "s.NO"() -> (w3882:string)
            n3043 = call <vilib>:"New Report.vi"("report type"=enum16{"Standard Report", "HTML"}."Standard Report") -> ("report out"=w3961:refnum<class "NI_report.lvclass">, "error out"=w3960:errorcluster)  [unwired: 13 in]
            n3044 = local read "TITTLE"() -> (w3913:string)
            n3045 = Concatenate Strings(w3938, w3881, w3882, w3938, w3916, w3911, w3938, w3915, w3912, w3938, w3917, w3914, w3938) -> (w3931:string)
            "test by" <- w3931
            n3046 = Number To Fractional String(number=w3937, width (-)=i16 6, precision (6)=i16 2) -> (F-format string=w3926:string)  [unwired: 1 in]
            n3047 = Number To Fractional String(number=w3936, width (-)=i16 6, precision (6)=i16 2) -> (F-format string=w3939:string)  [unwired: 1 in]
            n3048 = Number To Fractional String(number=w3952, width (-)=i16 6, precision (6)=i16 2) -> (F-format string=w3957:string)  [unwired: 1 in]
            n3049 = Number To Fractional String(number=w3941, width (-)=i16 6, precision (6)=i16 2) -> (F-format string=w3943:string)  [unwired: 1 in]
            n3050 = Number To Fractional String(number=w3927, width (-)=i16 6, precision (6)=i16 2) -> (F-format string=w3928:string)  [unwired: 1 in]
            n3051 = Number To Fractional String(number=w3940, width (-)=i16 6, precision (6)=i16 2) -> (F-format string=w3942:string)  [unwired: 1 in]
            n3052 = Number To Fractional String(number=w3923, width (-)=i16 6, precision (6)=i16 2) -> (F-format string=w3922:string)  [unwired: 1 in]
            n3053 = Number To Fractional String(number=w3919, precision (6)=i16 2) -> (F-format string=w3918:string)  [unwired: 2 in]
            n3054 = call-dynamic "Set Report Header Text.vi"("report in"=w3961, "center header text"=w3913, "error in (no error)"=w3960) -> ("report out"=w3932:refnum<class "NI_report.lvclass">, "error out"=w3933:errorcluster)  [unwired: 11 in]
            n3055 = Concatenate Strings(w3921, w3905, w3957, w3921, w3902, w3926, w3921, w3900, w3939, w3921, w3897, w3928, w3921, w3893, w3943, w3921, w3890, w3942, w3921, w3888, w3922, w3921, w3885, w3918) -> (w3909:string)
            "export 2" <- w3909
            n3056 = call-poly <vilib>:"Append Report Text.vi"("report in"=w3932, "text"=w3931, "error in (no error)"=w3933) -> ("report out"=w3935:refnum<class "NI_report.lvclass">, "error out"=w3934:errorcluster)  [unwired: 9 in, 2 out]
            n3057 = local read "test by"() -> (w3908:string)
            n3058 = local read "TITTLE"() -> (w3910:string)
            n3059 = call-poly <vilib>:"Append Report Text.vi"("report in"=w3935, "error in (no error)"=w3934) -> ("report out"=w3956:refnum<class "NI_report.lvclass">, "error out"=w3954:errorcluster)  [unwired: 10 in, 2 out]
            n3060 = Concatenate Strings(w3910, w3909, w3908) -> (→"output":string)
            n3061 = call-poly <vilib>:"Append Report Text.vi"("report in"=w3956, "text"=w3909, "error in (no error)"=w3954) -> ("report out"=w3955:refnum<class "NI_report.lvclass">, "error out"=w3953:errorcluster)  [unwired: 9 in, 2 out]
            n3062 = call-dynamic "Print Report.vi"("report in"=w3955, "printer name (default)"=w3963, "error in (no error)"=w3953) -> ("report out"=w3965:refnum<class "NI_report.lvclass">, "error out"=w3966:errorcluster)  [unwired: 11 in]
            n3063 = call-dynamic "Dispose Report.vi"("report in"=w3965, "error in (no error)"=w3966) -> ()  [unwired: 13 in, 1 out]
          }
        }
        n3064 = case shown="True" "Print 2" {
          frame False {
          }
          frame True {
            n3065 = flat-sequence {
              frame #0 {
                n3066 = local read "s.NO"() -> (→"s.NO 2":string)
                n3067 = Wait (ms)(milliseconds to wait=u32 20) -> ()  [unwired: 1 out]
                n3068 = local read "Sample ID  3"() -> (→"Sample ID  6":string)
                n3069 = local read "Sample ID  4"() -> (→"Sample ID  7":string)
                n3070 = local read "Sample ID"() -> (→"Sample ID  2":string)
                n3071 = local read "Tested by"() -> (→"Tested by 2":string)
                n3072 = local read "Test Date"() -> (→"Test Date 2":string)
                n3073 = local read "Humidity after test 3"() -> (→"Humidity after test 4":dbl)
